vi "findStringsNoImgs.vi"(2 "imgProperty":string, 3 "filenamesInput":string[](array[string])) -> (0 "noImgs":i32, 1 "filenamesOutput":string[](array[string]))   [LabVIEW 2015]
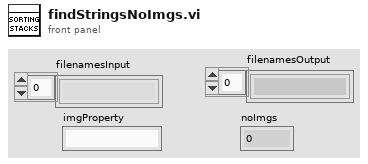
[diagram p1: front panel]
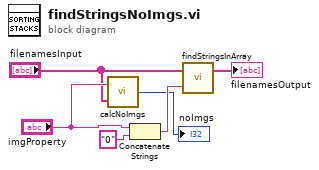
[diagram p0: block diagram]
diagram:
  n1 = call "calcNoImgs.vi"("filenames"="filenamesInput", "regExp"="imgProperty") -> ("noImgs"=→"noImgs":i32)
  n2 = Concatenate Strings("imgProperty", "0" ("string")) -> (w6:string)
  n3 = call "findStringsInArray.vi"("Regular expression"=w6, "1D string array"="filenamesInput") -> ("Matched array"=→"filenamesOutput":string[])  [unwired: 1 out]
